vi "Configure Switching Function.vi"(7 "function":u16(ring)=1 items=["1"=1, "2"=2, "3"=3, "4"=4, "5"=5, "6"=6], 8 "error in (no error)":errorcluster, 9 "thresholds":cluster{"lower":dbl, "upper":dbl}, 10 "mode":u16(ring)=1 items=["off", "on", "channel 1", "channel 2", "channel 3"], 11 "VGC in":refnum<class "PL Inficon VGC.lvclass">) -> (0 "error out":errorcluster, 1 "thresholds":cluster{"lower":dbl, "upper":dbl}, 2 "mode":u16(ring)=1 items=["off", "on", "channel 1", "channel 2", "channel 3"], 3 "VGC out":refnum<class "PL Inficon VGC.lvclass">)   [LabVIEW 2015, in "PL Inficon VGC.lvclass"]
doc: "Configures switching function."
uses:
  PL Inficon VGC.lvclass
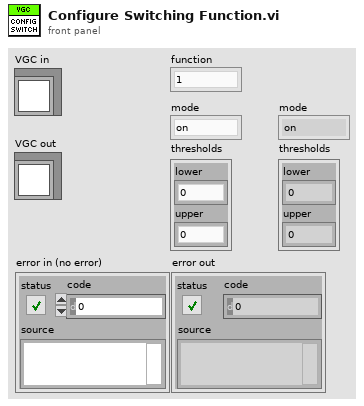
[diagram p1: front panel]
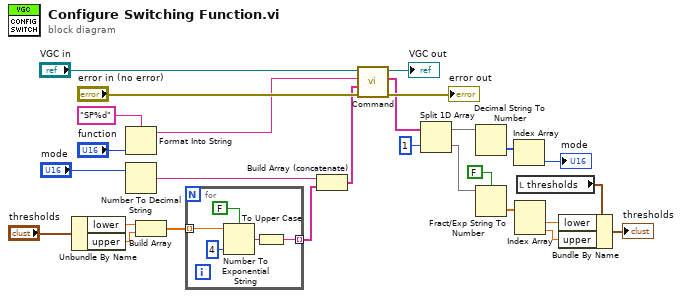
[diagram p0: block diagram]
diagram:
  n1 = Unbundle By Name("thresholds") -> ("lower"=w6:dbl, "upper"=w5:dbl)
  n2 = Format Into String(format string="SP%d", "function") -> (resulting string=w13:string)  [unwired: 2 in, 1 out]
  n3 = Number To Decimal String(number="mode") -> (decimal integer string=w16:string)  [unwired: 1 in]
  n4 = Build Array(w6, w5) -> (w9:dbl[])
  n5 = for {
    tunnel: w9 -> [w29] mode=indexing
    tunnel: [w28] -> w8 mode=indexing
    n6 = Number To Exponential String(number=w29, precision (6)=i16 4, 1:FALSE ("use system decimal point (T)")) -> (E-format string=w30:string)  [unwired: 1 in]
    n7 = To Upper Case(1:w30) -> (0:w28:string)
  }
  n8 = Build Array (concatenate)(w16, w8) -> (w12:string[])
  n9 = call "Command.vi"("error in (no error)"="error in (no error)", "parameters"=w12, "command"=w13, "VGC in"="VGC in") -> ("error out"=→"error out":errorcluster, "response data"=w22:string[], "VGC out"=→"VGC out":refnum<class "PL Inficon VGC.lvclass">)  [unwired: 5 in]
  n10 = Split 1D Array(array=w22, index=1) -> (first subarray=w20:string[], second subarray=w19:string[])
  n11 = Decimal String To Number(string=w20) -> (number=w11:i32[])  [unwired: 2 in, 1 out]
  n12 = Fract/Exp String To Number(use system decimal point (T)=FALSE, string=w19) -> (number=w18:dbl[])  [unwired: 2 in, 1 out]
  n13 = Index Array(array=w11) -> (element=→"mode":i32)  [unwired: 1 in]
  n14 = Index Array(array=w18) -> (element #1=w3:dbl, element #2=w2:dbl)  [unwired: 2 in]
  n15 = local read "thresholds"() -> (w4:cluster{"lower":dbl, "upper":dbl})
  n16 = Bundle By Name(cluster=w4, "lower"=w3, "upper"=w2) -> (→"thresholds":cluster{"lower":dbl, "upper":dbl})
